vi "MenuBuild.vi"(0 "Column in":refnum<class "Column.lvclass">, 1 "row type":T2, 3 "Clipboard":refnum<vi>, 5 "MenuRef In":refnum<k9>, 7 "Click Position":T1, 9 "Table CtlRef In":refnum<vi>, 11 "error in (no error)":errorcluster, 12 "withinSelection?":bool=TRUE, 14 "Button\n(Mouse Down?)":u16) -> (4 "Column out":refnum<class "Column.lvclass">, 6 "MenuRef Out":refnum<k9>, 10 "Table CtlRef Out":refnum<vi>, 15 "error out":errorcluster)   [LabVIEW 2013, in "Column.lvclass"]
doc: "Build shortcut (right-click) menu items for all columns in general. This VI is read-only w.r.t column data."
uses:
  Column.lvclass
  TypeDefs/RowType.ctl
  <vilib>/Utility/miscctls.llb/LVRowAndColumnTypeDef.ctl
panel:
  # "needed when providing multiple\nshortcut menus based on which\nmouse button clicked.\ne.g. LMenuCol override of\nMenuBuild method."
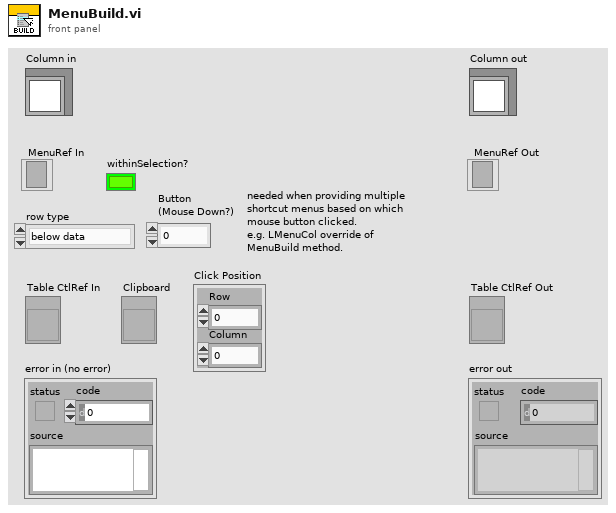
[diagram p1: front panel]
types:
  T1 = typedef "LVRowAndColumnTypeDef.ctl" = cluster{"Row":i32, "Column":i32}
  T2 = typedef "RowType.ctl" = enum16{"below data", "within data", "column header", "first row"}
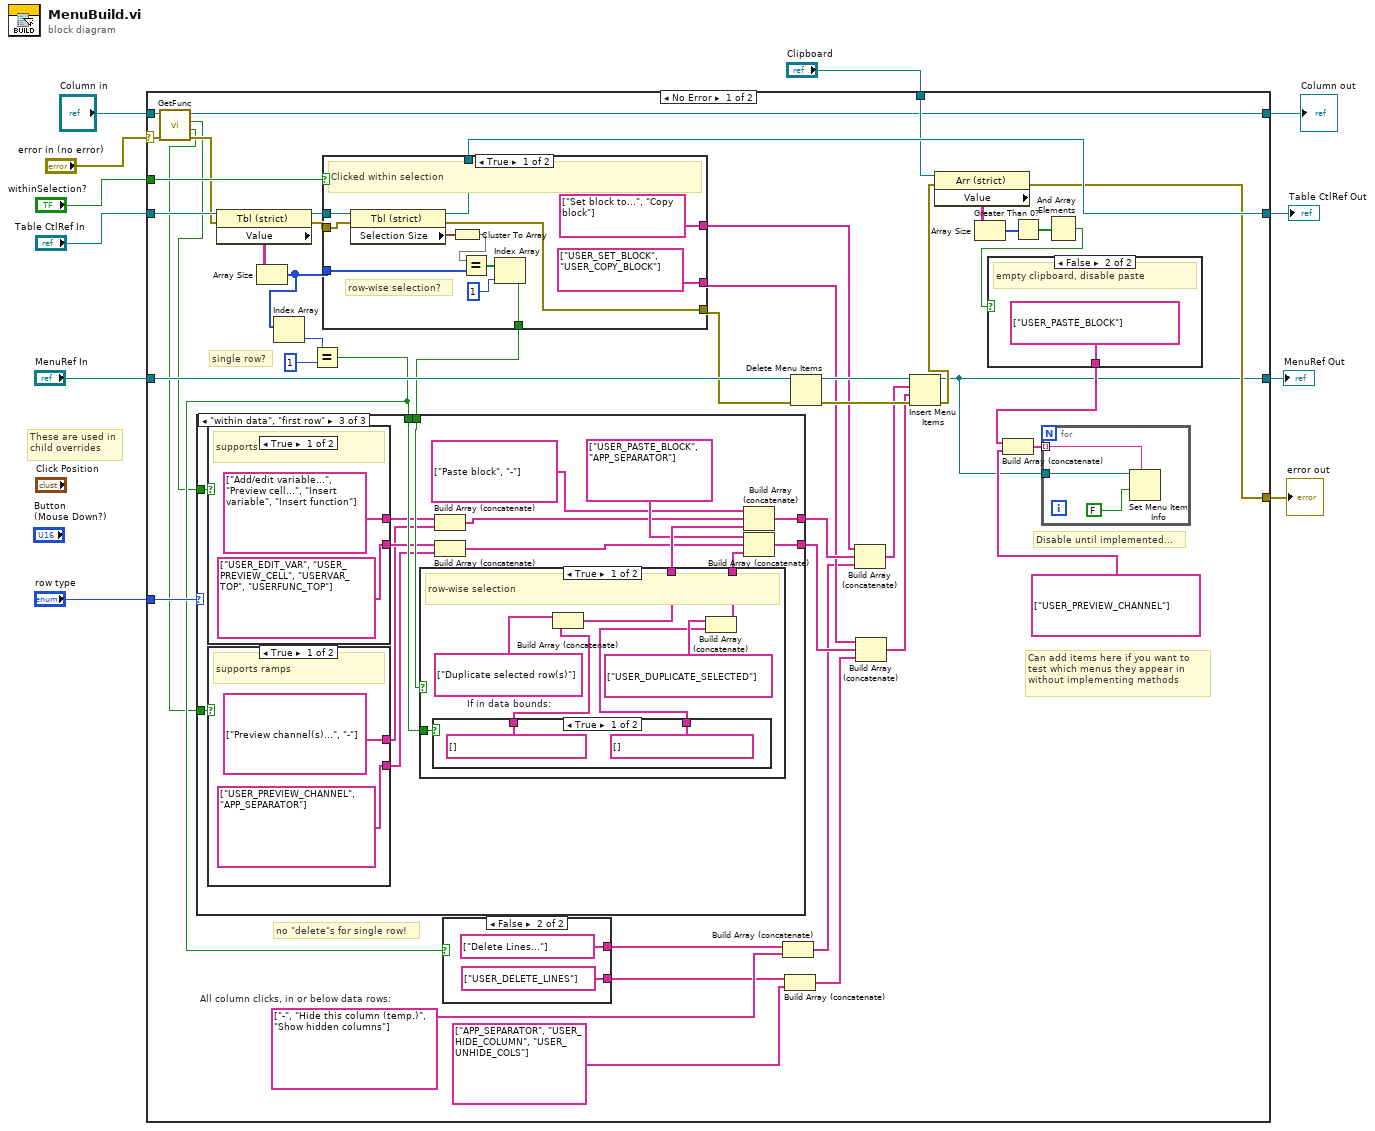
[diagram p0: block diagram]
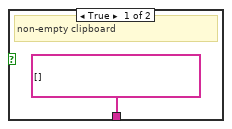
[diagram p2: hidden frame]
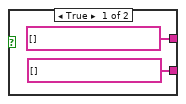
[diagram p3: hidden frame]
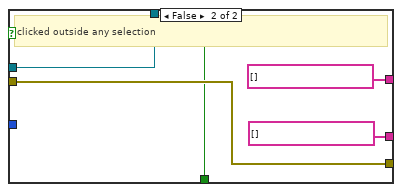
[diagram p4: hidden frame]
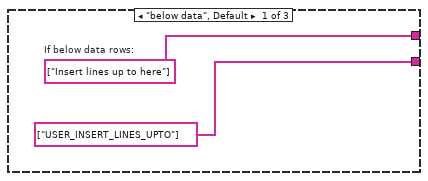
[diagram p5: hidden frame]
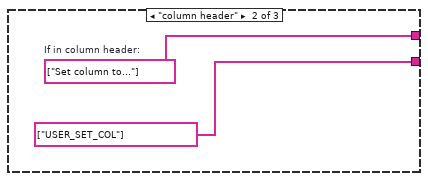
[diagram p6: hidden frame]
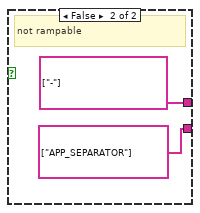
[diagram p7: hidden frame]
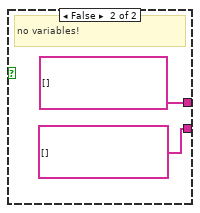
[diagram p8: hidden frame]
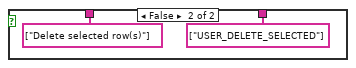
[diagram p9: hidden frame]
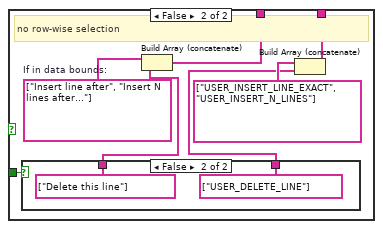
[diagram p10: hidden frame]
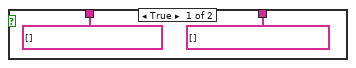
[diagram p11: hidden frame]
diagram:
  # "These are used in\nchild overrides"
  n1 = case shown="No Error" "error in (no error)" {
    selector: "error in (no error)" -> [w15 w133]
    tunnel: [w19 w133] -> w4
    tunnel: "Column in" -> [w17 w136]
    tunnel: [w16 w136] -> w11
    tunnel: "Table CtlRef In" -> [w42 w135]
    tunnel: "MenuRef In" -> [w50 w134]
    tunnel: [w18 w134] -> w8
    tunnel: [w48 w135] -> w7
    tunnel: "row type" -> [w49 _]
    tunnel: "withinSelection?" -> [w46 _]
    tunnel: "Clipboard" -> [w28 _]
    frame No Error {
      w34 = string[] ["-", "Hide this column (temp.)", "Show hidden columns"]  # All column clicks, in or below data rows:
      # "Can add items here if you want to \ntest which menus they appear in\nwithout implementing methods"
      # "Disable until implemented..."
      # "no \"delete\"s for single row!"
      # "single row?"
      n2 = call "GetFunc.vi"("error in (no error)"=w15, "Column in"=w17) -> ("error out"=w14:errorcluster, "isRampable?"=w12:bool, "isVariable?"=w13:bool, "Column out"=w16:refnum<class "Column.lvclass">)  [unwired: 5 in, 1 out]
      n3 = property class="Tbl (strict)"(reference=w42, error in=w14) -> (reference out=w41:refnum<vi>, error out=w40:errorcluster, "Value"=w39:string[][])
      n4 = Array Size(array=w39) -> (size(s)=w38:i32[])
      n5 = Index Array(array=w38) -> (element=w37:i32)  [unwired: 1 in]
      n6 = Equal?(x=w37, y=1) -> (x = y?=w29:bool)
      n7 = case shown="True" w46 {
        selector: w46 -> [_ w79]
        tunnel: [string[] ["Set block to...", "Copy block"] ("If within a selection:") string[] []] -> w44
        tunnel: [string[] ["USER_SET_BLOCK", "USER_COPY_BLOCK"] ("If within a selection:") string[] [] ("If within a selection:")] -> w43
        tunnel: w41 -> [w77 w81]
        tunnel: [w76 w81] -> w48
        tunnel: w40 -> [w71 w80]
        tunnel: [w70 w80] -> w47
        tunnel: [w67 w79] -> w45
        tunnel: w38 -> [w66 _]
        frame True {
          # "row-wise selection?"
          # "Clicked within selection"
          n8 = property class="Tbl (strict)"(reference=w77, error in=w71) -> (reference out=w76:refnum<vi>, error out=w70:errorcluster, "Selection Size"=w75:T1)
          n9 = Cluster To Array(cluster=w75) -> (array=w74:i32[])
          n10 = Equal?(x=w74, y=w66) -> (x = y?=w73:bool[])
          n11 = Index Array(array=w73, index=1) -> (element=w67:bool)
        }
        frame False {
          # "clicked outside any selection"
        }
      }
      n12 = case shown="\"within data\", \"first row\"" w49 {
        tunnel: [w84 w86 w102] -> w56
        tunnel: [string[] ["USER_INSERT_LINES_UPTO"] ("If below data rows:") string[] ["USER_SET_COL"] ("If below data rows:") w101] -> w55
        tunnel: w45 -> [_ _ w100]
        tunnel: w13 -> [_ _ w97]
        tunnel: w29 -> [_ _ w94]
        tunnel: w12 -> [_ _ w93]
        frame "below data", Default {
          w84 = string[] ["Insert lines up to here"]  # If below data rows:
        }
        frame "column header" {
          w86 = string[] ["Set column to..."]  # If in column header:
        }
        frame "within data", "first row" {
          n13 = case shown="True" w97 {
            tunnel: [string[] ["USER_EDIT_VAR", "USER_PREVIEW_CELL", "USERVAR_TOP", "USERFUNC_TOP"] ("If in data bounds:") string[] [] ("If in data bounds:")] -> w90
            tunnel: [string[] ["Add/edit variable...", "Preview cell...", "Insert variable", "Insert function"] ("If in data bounds:") string[] [] ("If in data bounds:")] -> w92
            frame True {
              # "supports variables"
            }
            frame False {
              # "no variables!"
            }
          }
          n14 = case shown="True" w93 {
            tunnel: [string[] ["USER_PREVIEW_CHANNEL", "APP_SEPARATOR"] ("If in data bounds:") string[] ["APP_SEPARATOR"] ("If in data bounds:")] -> w87
            tunnel: [string[] ["Preview channel(s)...", "-"] ("If in data bounds:") string[] ["-"] ("If in data bounds:")] -> w88
            frame True {
              # "supports ramps"
            }
            frame False {
              # "not rampable"
            }
          }
          n15 = case shown="True" w100 {
            tunnel: [w116 w127] -> w99
            tunnel: [w114 w125] -> w98
            tunnel: w94 -> [w111 w122]
            frame True {
              w115 = string[] ["Duplicate selected row(s)"]  # If in data bounds:
              # "row-wise selection"
              n16 = case shown="True" w111 {
                tunnel: [string[] [] string[] ["Delete selected row(s)"]] -> w113
                tunnel: [string[] [] string[] ["USER_DELETE_SELECTED"]] -> w112
                frame True {
                }
                frame False {
                }
              }
              n17 = Build Array (concatenate)(w115, w113) -> (w114:string[])
              n18 = Build Array (concatenate)(string[] ["USER_DUPLICATE_SELECTED"] ("If in data bounds:"), w112) -> (w116:string[])
            }
            frame False {
              w126 = string[] ["Insert line after", "Insert N lines after..."]  # If in data bounds:
              # "no row-wise selection"
              n19 = case shown="False" w122 {
                tunnel: [string[] [] string[] ["Delete this line"]] -> w124
                tunnel: [string[] [] string[] ["USER_DELETE_LINE"]] -> w123
                frame True {
                }
                frame False {
                }
              }
              n20 = Build Array (concatenate)(w126, w124) -> (w125:string[])
              n21 = Build Array (concatenate)(string[] ["USER_INSERT_LINE_EXACT", "USER_INSERT_N_LINES"] ("If in data bounds:"), w123) -> (w127:string[])
            }
          }
          n22 = Build Array (concatenate)(w92, w88) -> (w91:string[])
          n23 = Build Array (concatenate)(w90, w87) -> (w89:string[])
          n24 = Build Array (concatenate)(string[] ["Paste block", "-"] ("If within a selection:"), w91, w98) -> (w102:string[])
          n25 = Build Array (concatenate)(string[] ["USER_PASTE_BLOCK", "APP_SEPARATOR"] ("If within a selection:"), w89, w99) -> (w101:string[])
        }
      }
      n26 = case shown="False" w29 {
        tunnel: [string[] [] string[] ["Delete Lines..."]] -> w35
        tunnel: [string[] [] string[] ["USER_DELETE_LINES"]] -> w32
        frame True {
        }
        frame False {
        }
      }
      n27 = Build Array (concatenate)(w35, w34) -> (w33:string[])
      n28 = Build Array (concatenate)(w32, string[] ["APP_SEPARATOR", "USER_HIDE_COLUMN", "USER_UNHIDE_COLS"] ("If within a selection:")) -> (w30:string[])
      n29 = Delete Menu Items(6:w47, 9:w50) -> (0:w54:errorcluster, 3:w53:refnum<k9>)  [unwired: 2 in]
      n30 = Build Array (concatenate)(w44, w56, w33) -> (w52:string[])
      n31 = Build Array (concatenate)(w43, w55, w30) -> (w51:string[])
      n32 = Insert Menu Items(6:w54, 7:w51, 8:w52, 9:w53) -> (0:w20:errorcluster, 3:w18:refnum<k9>)  [unwired: 2 in, 1 out]
      n33 = property class="Arr (strict)"(reference=w28, error in=w20) -> (error out=w19:errorcluster, "Value"=w27:string[][])  [unwired: 1 out]
      n34 = Array Size(array=w27) -> (size(s)=w26:i32[])
      n35 = Greater Than 0?(x=w26) -> (x > 0?=w25:bool[])
      n36 = And Array Elements(Boolean array=w25) -> (logical AND=w21:bool)
      n37 = case shown="False" w21 {
        tunnel: [string[] [] ("If within a selection:") string[] ["USER_PASTE_BLOCK"] ("If within a selection:")] -> w24
        frame True {
          # "non-empty clipboard"
        }
        frame False {
          # "empty clipboard, disable paste"
        }
      }
      n38 = Build Array (concatenate)(w24, string[] ["USER_PREVIEW_CHANNEL"] ("If within a selection:")) -> (w22:string[])
      n39 = for {
        tunnel: w22 -> [w59] mode=indexing
        tunnel: w18 -> [w61]
        n40 = Set Menu Item Info(7:w59, 9:FALSE ("enabled"), 11:w61) -> ()  [unwired: 4 in, 2 out]
      }
    }
    frame Error {
    }
  }
  "error out" <- w4
  "Column out" <- w11
  "MenuRef Out" <- w8
  "Table CtlRef Out" <- w7
